vi "testPinvTruncate.vi"(8 "error in (no error)":errorcluster) -> (0 "error out":errorcluster)   [LabVIEW 2016]
doc: "Test to do the pseudo inverse with the truncation based on the threshold."
uses:
  <vilib>/Analysis/baseanly.llb/Real A x B.vi
  <vilib>/Analysis/_algsub.llb/Real Matrix Trace.vi
  <vilib>/Analysis/Matrix/Numeric/Conversions/Array To Matrix - RA2.vi
  <vilib>/addons/_JKI Toolkits/Caraya/classes/Assert/Assert.lvclass
  <vilib>/addons/_JKI Toolkits/Caraya/classes/Test/Test.lvclass
  MatOper/MatOper.lvclass
  <vilib>/Analysis/Matrix/NI_Matrix.lvlib
  <vilib>/Analysis/NI_AALBase.lvlib
  <vilib>/Analysis/NI_AALPro.lvlib
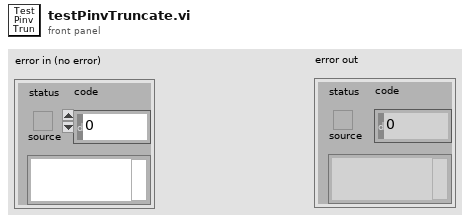
[diagram p1: front panel]
types:
  T1 = typedef "NI_Matrix.lvlib/RealMatrix.ctl" = dbl[][]
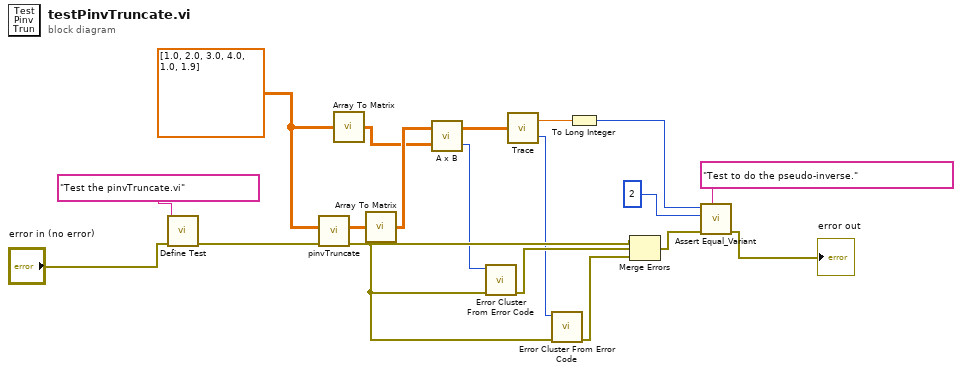
[diagram p0: block diagram]
diagram:
  w15 = dbl[][] [[1.0, 2.0], [3.0, 4.0], [1.0, 1.9]]
  n1 = call <vilib>:"Define Test.vi"("error in (no error)"="error in (no error)", "Label (VI Title)"="Test the pinvTruncate.vi") -> ("error out"=w16:errorcluster)  [unwired: 9 in]
  n2 = call "pinvTruncate.vi"("error in (no error)"=w16, "Matrix A"=w15) -> ("error out"=w7:errorcluster, "Truncated Pinv A"=w14:dbl[][])  [unwired: 7 in, 1 out]
  n3 = call-poly <vilib>:"Array To Matrix.vi"("Real 2D Array"=w15) -> ("Real Matrix"=w11:T1)
  n4 = call-poly <vilib>:"Array To Matrix.vi"("Real 2D Array"=w14) -> ("Real Matrix"=w12:T1)
  n5 = call-poly <vilib>:"A x B.vi"("B"=w11, "A"=w12) -> ("error"=w6:i32, "A x B"=w13:T1)
  n6 = call <vilib>:"Error Cluster From Error Code.vi"("error in (no error)"=w7, "error code (0)"=w6) -> ("error out"=w5:errorcluster)  [unwired: 7 in]
  n7 = call-poly <vilib>:"Trace.vi"("Input Matrix"=w13) -> ("trace"=w10:dbl, "error"=w4:i32)
  n8 = call <vilib>:"Error Cluster From Error Code.vi"("error in (no error)"=w7, "error code (0)"=w4) -> ("error out"=w3:errorcluster)  [unwired: 7 in]
  n9 = To Long Integer(number=w10) -> (32bit integer=w9:i32)
  n10 = Merge Errors(w7, w5, w3) -> (w2:errorcluster)
  n11 = call <vilib>:"Assert Equal_Variant.vi"("Label"="Test to do the pseudo-inverse.", "error in (no error)"=w2, "Y"=2, "X"=w9) -> ("error out"=→"error out":errorcluster)  [unwired: 7 in]
